vi "Floor_Negative16.vi"(10 "Baseline U16":u16, 11 "Input Value":i16) -> (3 "Output Value":u16)   [LabVIEW 2012]
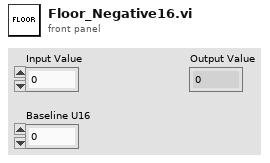
[diagram p1: front panel]
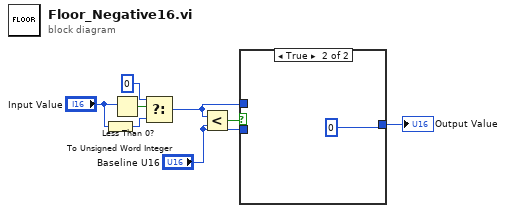
[diagram p0: block diagram]
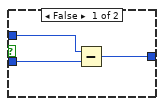
[diagram p2: hidden frame]
diagram:
  n1 = To Unsigned Word Integer(number="Input Value") -> (unsigned 16bit integer=w4:u16)
  n2 = Less Than 0?(x="Input Value") -> (x < 0?=w5:bool)
  n3 = Select(t=u16 0, s=w5, f=w4) -> (s? t:f=w2:u16)
  n4 = Less?(x=w2, y="Baseline U16") -> (x < y?=w8:bool)
  n5 = case shown="True" w8 {
    tunnel: w2 -> [w11 _]
    tunnel: "Baseline U16" -> [w10 _]
    tunnel: [w9 u16 0] -> w6
    frame False {
      n6 = Subtract(x=w11, y=w10) -> (x-y=w9:u16)
    }
    frame True {
    }
  }
  "Output Value" <- w6
